vi "Evaluation.vi"(6 "ToEvaluate in":refnum<data-value>, 8 "error in (no error)":errorcluster, 10 "Parents G":dbl, 11 "MultiTree in":refnum<class "MultiTree.lvclass">) -> (0 "error out":errorcluster, 1 "H":dbl, 2 "G":dbl, 3 "MultiTree out":refnum<class "MultiTree.lvclass">, 4 "ToEvaluate out":refnum<data-value>)   [LabVIEW 2014, in "MultiTree.lvlib" / "MultiTree.lvclass"]
uses:
  <userlib>/AdvancedDataStructures/ClassBased/MultiTree/MultiTree.lvclass
  <userlib>/AdvancedDataStructures/ClassBased/MultiTreeNode/MultiTreeNode.lvclass
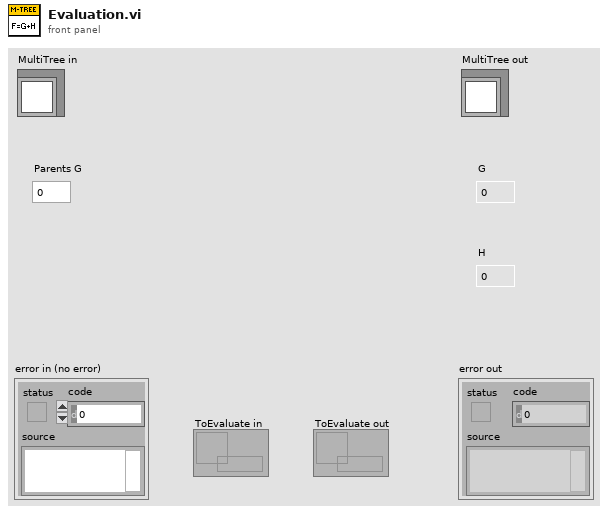
[diagram p1: front panel]
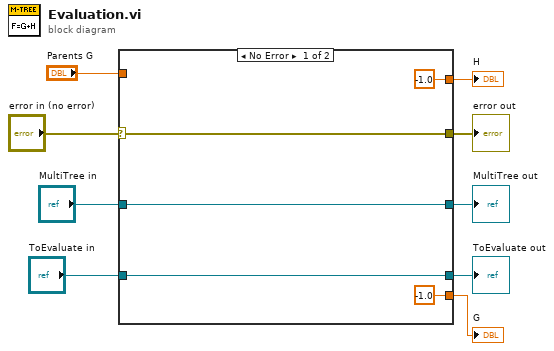
[diagram p0: block diagram]
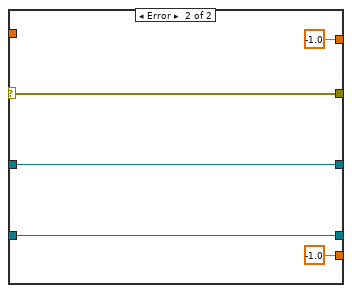
[diagram p2: hidden frame]
diagram:
  n1 = case shown="No Error" "error in (no error)" {
    selector: "error in (no error)" -> [w13 w19]
    tunnel: [w13 w19] -> w8
    tunnel: [w14 w18] -> w6
    tunnel: "MultiTree in" -> [w14 w18]
    tunnel: [w12 w17] -> w5
    tunnel: "ToEvaluate in" -> [w12 w17]
    tunnel: "Parents G" -> [_ _]
    tunnel: [-1.0 -1.0] -> w2
    tunnel: [-1.0 -1.0] -> w1
    frame No Error {
    }
    frame Error {
    }
  }
  "error out" <- w8
  "MultiTree out" <- w6
  "ToEvaluate out" <- w5
  "G" <- w2
  "H" <- w1
